vi "Save_compile_variables.vi"(0 "frN":dbl format="%.2f", 1 "TensionD Pelvis":dbl[](array[numeric]), 2 "A Pelvic Matrix":T1, 5 "DesiredFM":dbl[](array[numeric]), 7 "DesiredFMPel":dbl[](array[numeric]), 9 "AcTension(all)":dbl[](array[numeric]), 11 "TensionD Trunk":dbl[](array[numeric]), 12 "TensionD knees":dbl[](array[numeric]), 13 "A Trunk Matrix":T1) -> (15 "Save Output array":dbl[](array[numeric]))   [LabVIEW 2017]
uses:
  <vilib>/Analysis/Matrix/Datatypes/RealMatrix.ctl
  <vilib>/Analysis/Matrix/NI_Matrix.lvlib
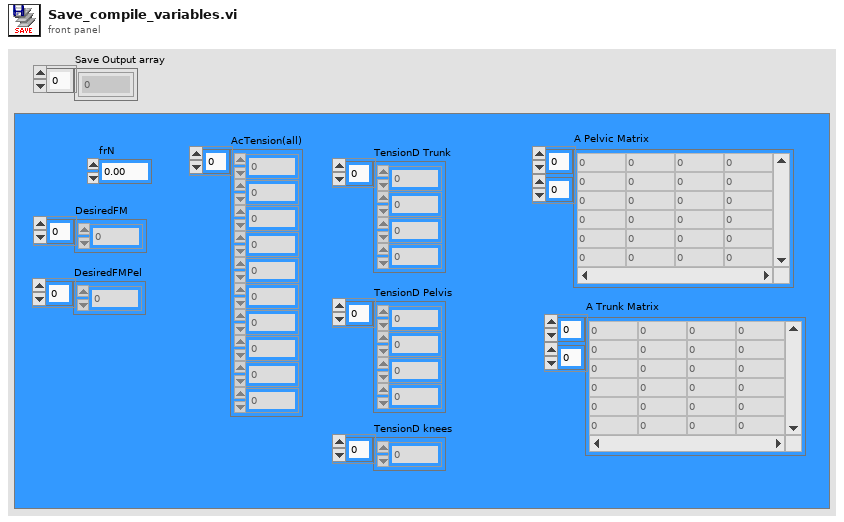
[diagram p1: front panel]
types:
  T1 = typedef "NI_Matrix.lvlib/RealMatrix.ctl" = dbl[][]
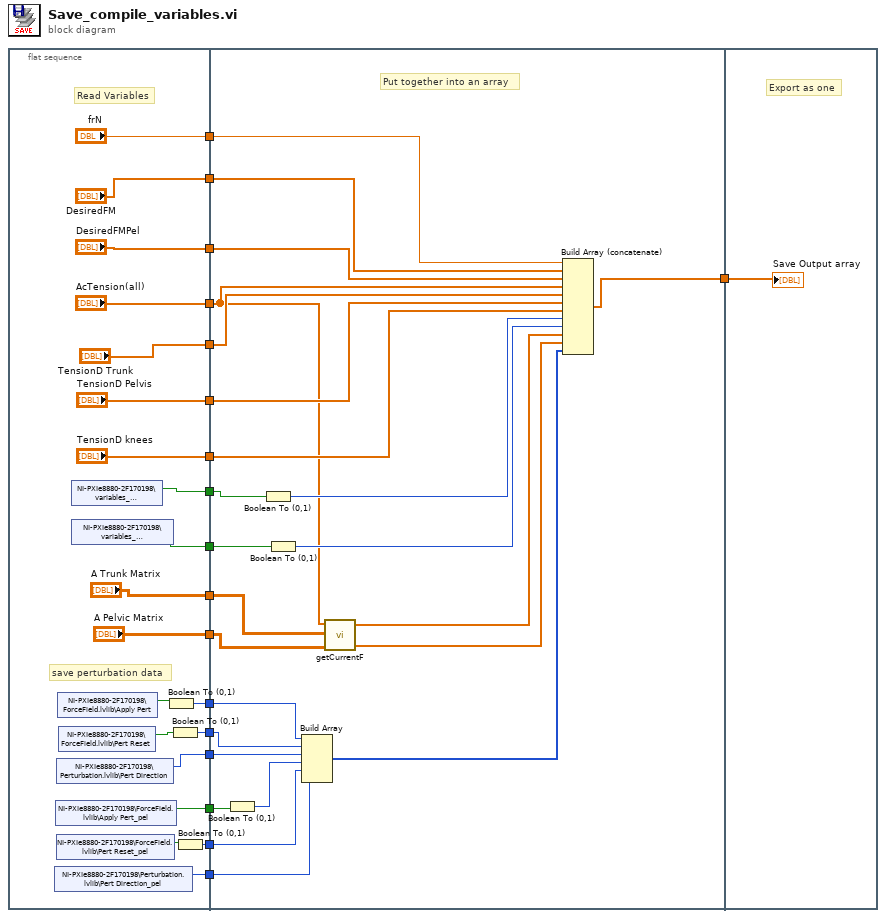
[diagram p0: block diagram]
diagram:
  n1 = flat-sequence {
    tunnel: ["frN"] -> w18
    tunnel: ["DesiredFM"] -> w17
    tunnel: ["DesiredFMPel"] -> w16
    tunnel: ["AcTension(all)"] -> w15
    tunnel: ["TensionD Trunk"] -> w14
    tunnel: ["TensionD Pelvis"] -> w13
    tunnel: ["TensionD knees"] -> w12
    tunnel: [w31] -> w11
    tunnel: [w30] -> w10
    tunnel: ["A Trunk Matrix"] -> w8
    tunnel: ["A Pelvic Matrix"] -> w7
    tunnel: [w27] -> w6
    tunnel: [w26] -> w5
    tunnel: [w24] -> w4
    tunnel: [w21] -> w3
    tunnel: [w20] -> w2
    tunnel: [w19] -> w1
    tunnel: w18 -> [w62]
    tunnel: w17 -> [w61]
    tunnel: w16 -> [w60]
    tunnel: w15 -> [w52]
    tunnel: w14 -> [w59]
    tunnel: w13 -> [w58]
    tunnel: w12 -> [w57]
    tunnel: w11 -> [w56]
    tunnel: w10 -> [w54]
    tunnel: [w39] -> w9
    tunnel: w8 -> [w50]
    tunnel: w7 -> [w51]
    tunnel: w6 -> [w47]
    tunnel: w5 -> [w46]
    tunnel: w4 -> [w44]
    tunnel: w3 -> [w43]
    tunnel: w2 -> [w42]
    tunnel: w1 -> [w41]
    tunnel: w9 -> [w63]
    frame #0 {
      # "save perturbation data"
      # "Read Variables"
      n2 = shared-variable "NI-PXIe8880-2F170198\\Perturbation.lvlib\\Pert Direction_pel"() -> (w19:i16)  [unwired: 1 in, 1 out]
      n3 = shared-variable "NI-PXIe8880-2F170198\\ForceField.lvlib\\Apply Pert_pel"() -> (w26:bool)  [unwired: 1 in, 1 out]
      n4 = shared-variable "NI-PXIe8880-2F170198\\Perturbation.lvlib\\Pert Direction"() -> (w27:i16)  [unwired: 1 in, 1 out]
      n5 = shared-variable "NI-PXIe8880-2F170198\\ForceField.lvlib\\Pert Reset_pel"() -> (w25:bool)  [unwired: 1 in, 1 out]
      n6 = shared-variable "NI-PXIe8880-2F170198\\ForceField.lvlib\\Apply Pert"() -> (w22:bool)  [unwired: 1 in, 1 out]
      n7 = shared-variable "NI-PXIe8880-2F170198\\ForceField.lvlib\\Pert Reset"() -> (w23:bool)  [unwired: 1 in, 1 out]
      n8 = shared-variable "NI-PXIe8880-2F170198\\variables_ForceModeUsingVicon - networkPublished.lvlib\\Error_QP"() -> (w31:bool)  [unwired: 1 in, 1 out]
      n9 = shared-variable "NI-PXIe8880-2F170198\\variables_ForceModeUsingVicon - networkPublished.lvlib\\Error_QP_2"() -> (w30:bool)  [unwired: 1 in, 1 out]
      n10 = Boolean To (0,1)(Boolean=w22) -> (0, 1=w21:i16)
      n11 = Boolean To (0,1)(Boolean=w23) -> (0, 1=w20:i16)
      n12 = Boolean To (0,1)(Boolean=w25) -> (0, 1=w24:i16)
    }
    frame #1 {
      # "Put together into an array"
      n13 = Boolean To (0,1)(Boolean=w46) -> (0, 1=w45:i16)
      n14 = Boolean To (0,1)(Boolean=w56) -> (0, 1=w55:i16)
      n15 = Boolean To (0,1)(Boolean=w54) -> (0, 1=w53:i16)
      n16 = Build Array(w43, w42, w47, w45, w44, w41) -> (w40:i16[])
      n17 = call "getCurrentF.vi"("AcTension(all)"=w52, "A Trunk Matrix"=w50, "A Pelvic Matrix"=w51) -> ("ActF Trunk"=w49:dbl[], "ActF Pelvis"=w48:dbl[])  [unwired: 3 in]
      n18 = Build Array (concatenate)(w62, w61, w60, w52, w59, w58, w57, w55, w53, w49, w48, w40) -> (w39:dbl[])
    }
    frame #2 {
      # "Export as one"
      "Save Output array" <- w63
    }
  }
